vi "Read DM-SetPower-Command-Arguments.vi"(8 "error in (no error)":errorcluster, 11 "DM-SetPower-Command in":refnum<class "DM-SetPower-Command.lvclass">) -> (0 "error out":errorcluster, 2 "DM-SetPower-Command-In":T1 {"Power" scale=-1.0..1.0}, 3 "DM-SetPower-Command out":refnum<class "DM-SetPower-Command.lvclass">)   [LabVIEW 2013, in "DM-SetPower-Command.lvclass"]
uses:
  DM-SetPower-Command.lvclass
  DM-SetPower-Command-Arguments.ctl
  DM-SetPower-Command.lvclass/DM-SetPower-Command.ctl
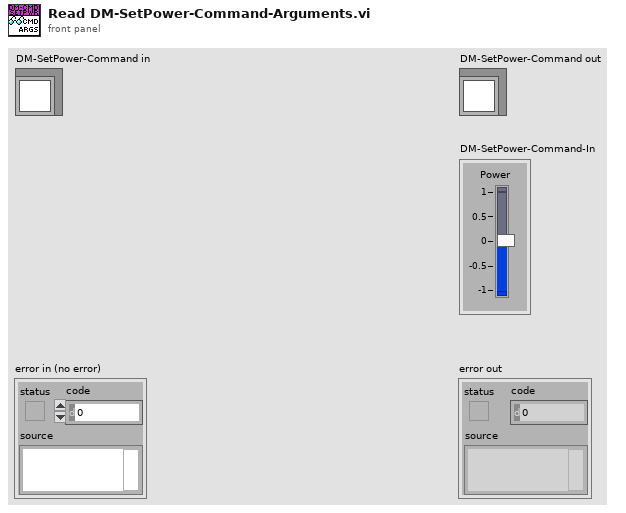
[diagram p1: front panel]
types:
  T1 = typedef "DM-SetPower-Command.lvclass/DM-SetPower-Command-Arguments.ctl" = cluster{"Power":dbl}
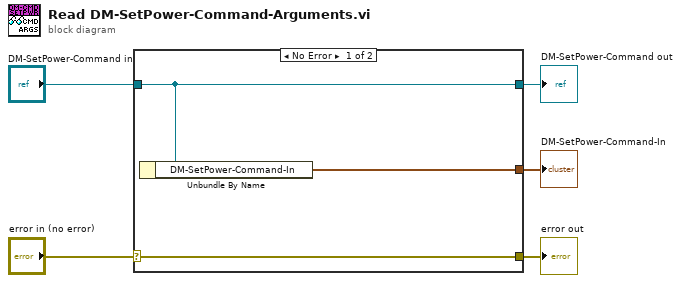
[diagram p0: block diagram]
diagram:
  n1 = case shown="No Error" "error in (no error)" {
    selector: "error in (no error)" -> [w8 w9]
    tunnel: [w8 w9] -> w4
    tunnel: [w7 w10] -> w2
    tunnel: "DM-SetPower-Command in" -> [w7 w10]
    tunnel: [w6 _] -> w1
    frame No Error {
      n2 = Unbundle By Name(w7) -> ("DM-SetPower-Command-In"=w6:T1)
    }
    frame Error {
    }
  }
  "error out" <- w4
  "DM-SetPower-Command out" <- w2
  "DM-SetPower-Command-In" <- w1
